vi "PH_Beamline_Chief.ProcPeriodic.vi"(0 "i ref in":refnum<vi>, 3 "ms timeout (100)":i32=100, 5 "error in (no error)":errorcluster) -> (14 "i ref out":refnum<vi>, 17 "timed out":bool, 19 "error out":errorcluster)   [LabVIEW 2014, in "PH_Beamline_Chief.lvlib"]
doc: "This method serves to periodically do things like reading values from the HW. Methods that should be executed periodically should be called from THIS methode. Add code here."
uses:
  PH_Beamline_Chief.lvlib
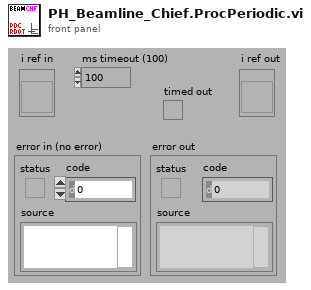
[diagram p1: front panel]
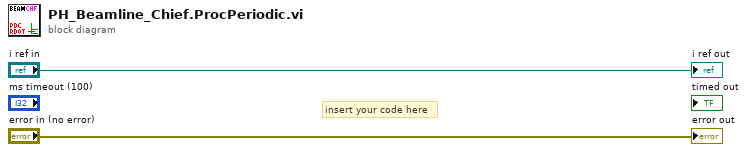
[diagram p0: block diagram]
diagram:
  # "insert your code here"
  "error out" <- "error in (no error)"
  "i ref out" <- "i ref in"
